vi "Main.vi"(11 "Module Admin":refnum<class "Delacor_lib_QMH_Module Admin.lvclass">) -> ()   [LabVIEW 2024, in "FunctionGenerator.lvlib"]
doc: "This template is based off of the Queued Message Handler design pattern and the Queued Message Handler project template that ships with LabVIEW.\n\nThe main difference is that the queue is private to this module and communication between modules is performed via Broadcast and Request events.\n\nRequest events are wrapped in public API methods and are handled in the Event Handling Loop (EHL) of this VI. Any module can register for Broadcast events sent by this module. The EHL generates messages based on user interface actions.\n\nThe Message Handling Loop (MHL) processes messages generated by the EHL, or by other messages. The messages are string values, so new messages can be added easily to the Message Cases case structure in the MHL. Each message cluster can also provide an optional value for Message Data, which is a variant that can be converted to whatever message-specific data is required.\n_____\nBased on DQMH Dev Tools: Project Template 7.1.0.1503."
uses:
  FunctionGenerator.lvlib
  <vilib>/Delacor/Delacor QMH/Libraries/Module Admin_class/Delacor_lib_QMH_Module Admin.lvclass
  Module Data--cluster.ctl
  <vilib>/Delacor/Delacor QMH/Libraries/Message Queue_class/Delacor_lib_QMH_Message Queue.lvclass/Delacor_lib_QMH_Message Queue.ctl
  Stop Argument--cluster.ctl
  <vilib>/Delacor/Delacor QMH/Libraries/Module Admin_class/Delacor_lib_QMH_Module Admin.lvclass/Delacor_lib_QMH_Module Admin.ctl
  Set Signal Type Argument--cluster.ctl
  Set Amplitude Argument--cluster.ctl
  Set Frecuency Argument--cluster.ctl
  Set Offset Argument--cluster.ctl
  Get Waveform Argument--cluster.ctl
  Get Waveform (Reply Payload)--cluster.ctl
  <vilib>/Utility/miscctls.llb/LVPointTypeDef.ctl
  <vilib>/Delacor/Delacor QMH/Libraries/Message Queue_class/Delacor_lib_QMH_Enqueue Message (Single).vi
  <vilib>/Delacor/Delacor QMH/Libraries/Module Admin_class/Delacor_lib_QMH_Get External Launch.vi
  <vilib>/Delacor/Delacor QMH/Libraries/Message Queue_class/Delacor_lib_QMH_Message Queue.lvclass
  <vilib>/measure/NI_MABase.lvlib
panel:
  out "error out":errorcluster
  out "Status":string
  in  "Simulate MHL Error":bool
  in  "Simulate EHL Error":bool
  # "Other processes communicate with this Module via its Public API (wrappers for its Request Events).\n\nThis Module communicates with other processes via its Broadcast Events.\nAny process that wants to receive these messages can register for this module's Broadcast events."
  # "This template is for the DQMH framework. See the block diagram for more information on how to use this template."
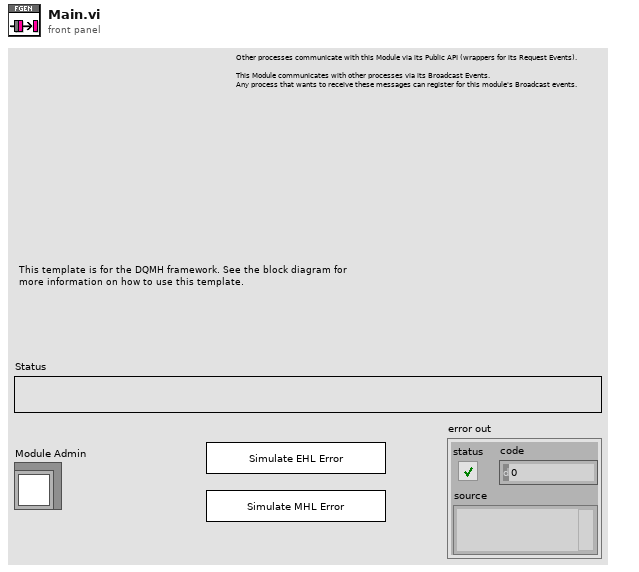
[diagram p1: front panel]
types:
  T1 = typedef "FunctionGenerator.lvlib/Request Events--cluster.ctl" = cluster{"Stop Module":refnum<user-event>, "Show Panel":refnum<user-event>, "Hide Panel":refnum<user-event>, "Get Module Execution Status":refnum<user-event>, "Show Diagram":refnum<user-event>, "Set Signal Type":refnum<user-event>, "Set Amplitude":refnum<user-event>, "Set Frecuency":refnum<user-event>, "Set Offset":refnum<user-event>, "Get Waveform":refnum<user-event>}
  T2 = typedef "FunctionGenerator.lvlib/Module Data--cluster.ctl" = cluster{"Status":string, "signal type":enum16{"Sine Wave", "Triangle Wave", "Square Wave", "Sawtooth Wave"}, "Amplitude":dbl, "Frecuency":dbl, "Offset":dbl}
  T3 = enum32{"invalid lock state", "Not Locked", "Locked (No Password)", "Password-protected"}
  T4 = typedef "FunctionGenerator.lvlib/Stop Argument--cluster.ctl" = cluster{"Origin":string, "Exit via Stop Module Req?":bool, "Wait for Module to stop?":bool}
  T5 = typedef "FunctionGenerator.lvlib/Set Signal Type Argument--cluster.ctl" = cluster{"signal type":enum16{"Sine Wave", "Triangle Wave", "Square Wave", "Sawtooth Wave"}}
  T6 = typedef "FunctionGenerator.lvlib/Set Amplitude Argument--cluster.ctl" = cluster{"Amplitude":dbl}
  T7 = typedef "FunctionGenerator.lvlib/Set Frecuency Argument--cluster.ctl" = cluster{"Frecuency":dbl}
  T8 = typedef "FunctionGenerator.lvlib/Set Offset Argument--cluster.ctl" = cluster{"Offset":dbl}
  T9 = typedef "FunctionGenerator.lvlib/Get Waveform Argument--cluster.ctl" = cluster{"Wait Notifier":refnum<notifier>, "wait for reply":bool}
  T10 = typedef "LVPointTypeDef.ctl" = cluster{"Horizontal":i16, "Vertical":i16}
  T11 = enum32{"Invalid", "Standard", "Closed", "Hidden", "Minimized", "Maximized"}
  T12 = typedef "FunctionGenerator.lvlib/Get Waveform (Reply Payload)--cluster.ctl" = cluster{"Waveform":waveform(dbl), "error":errorcluster}
  T13 = enum16{"Sine Wave", "Triangle Wave", "Square Wave", "Sawtooth Wave"}
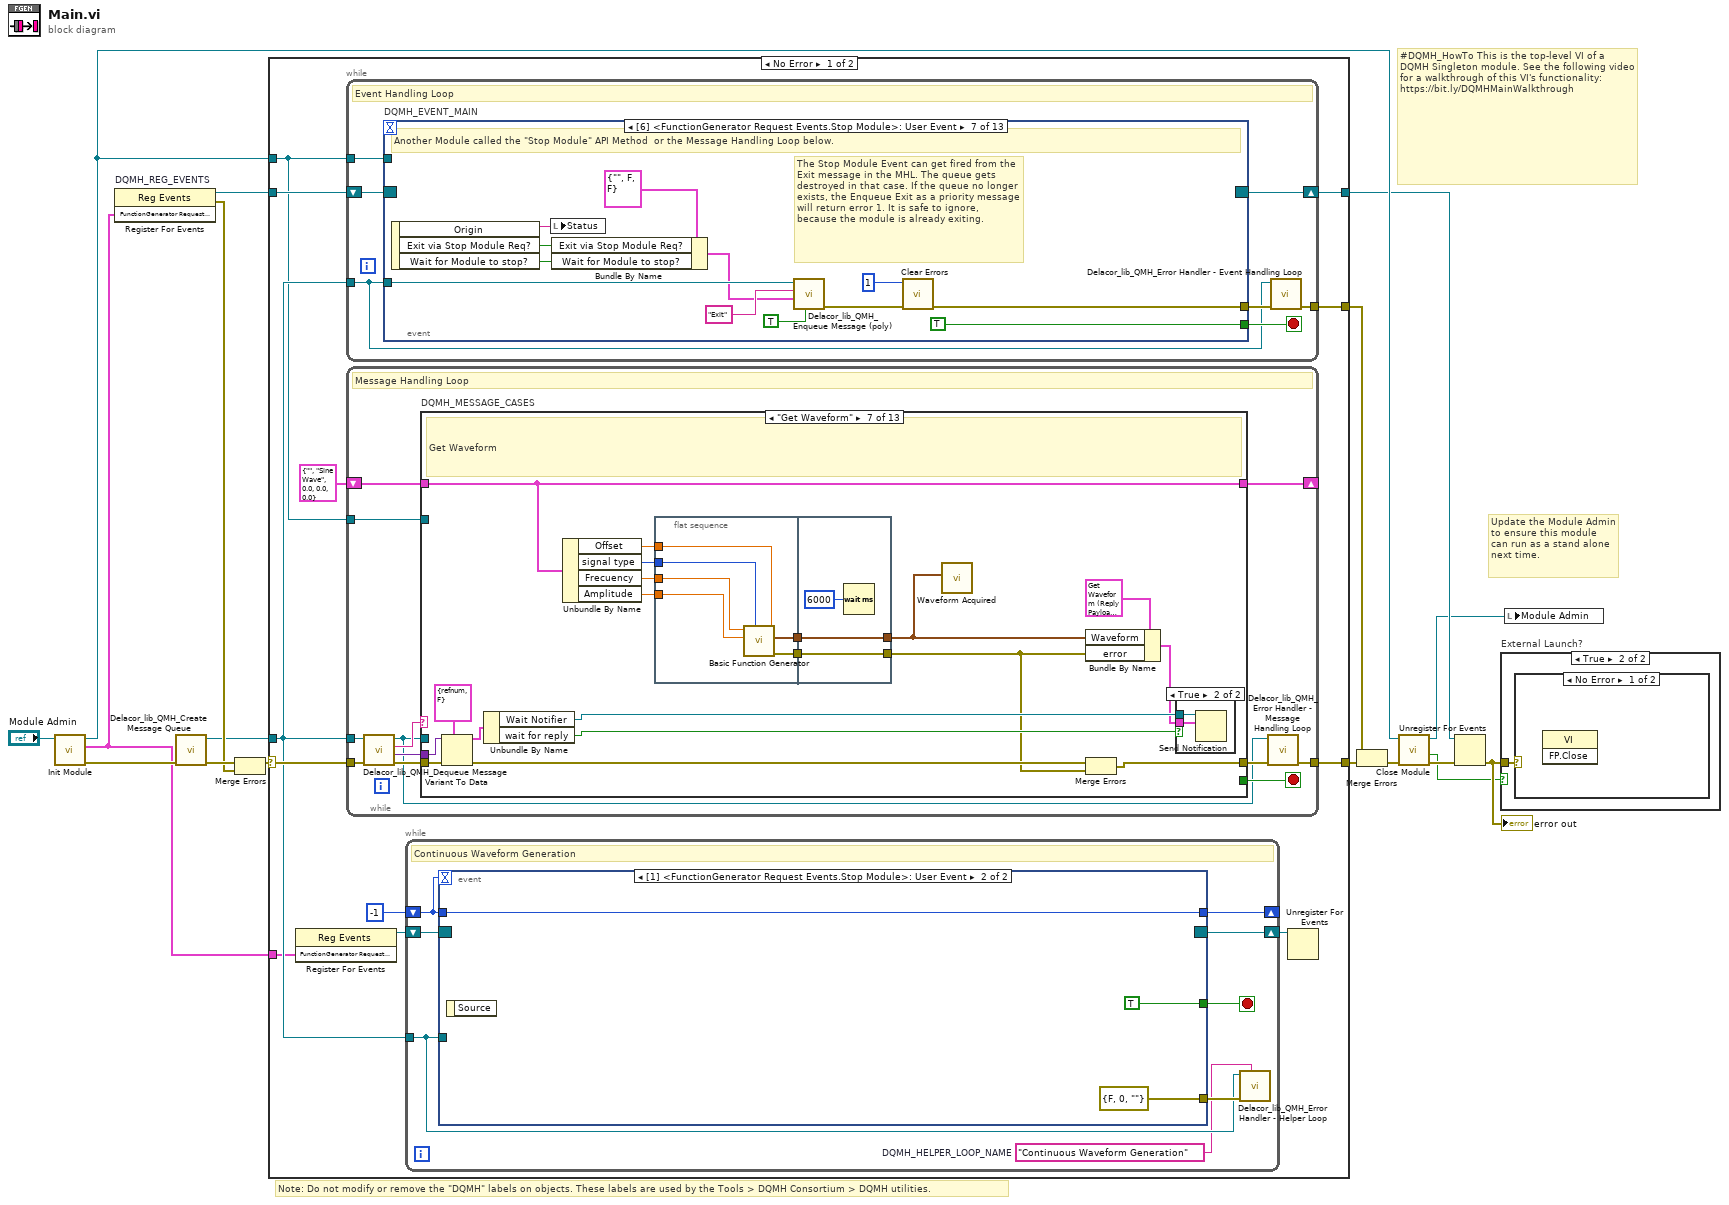
[diagram p0: block diagram]
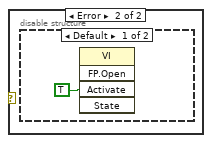
[diagram p3: hidden frame]
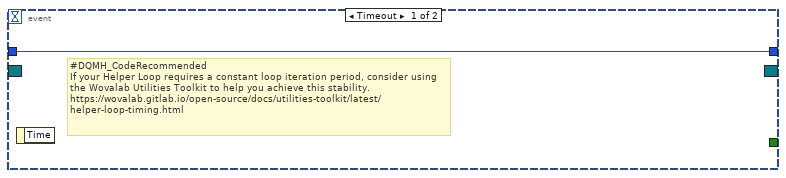
[diagram p5: hidden frame]
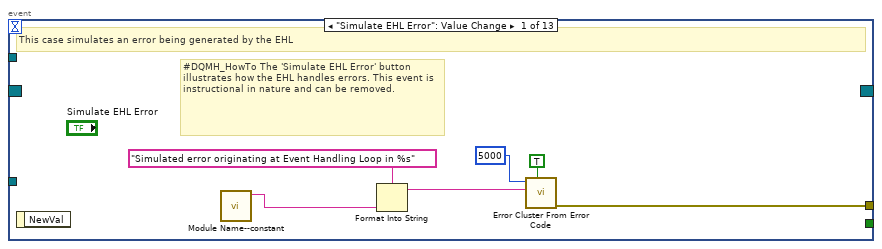
[diagram p6: hidden frame]
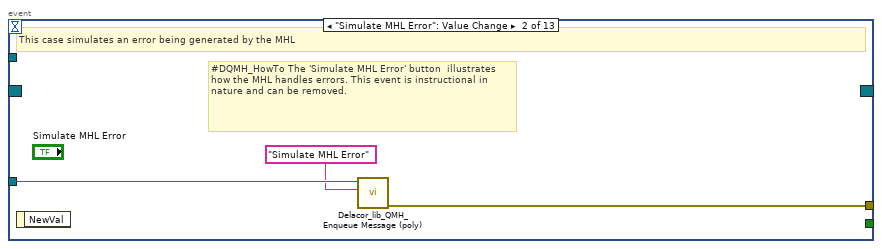
[diagram p7: hidden frame]
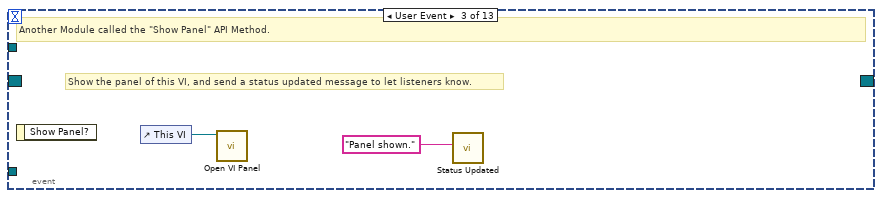
[diagram p8: hidden frame]
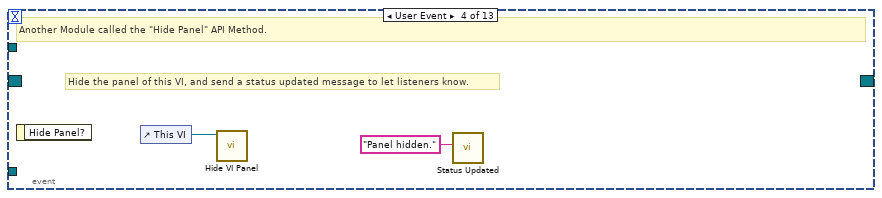
[diagram p9: hidden frame]
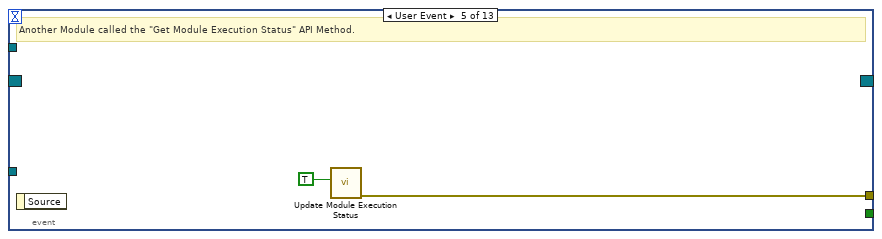
[diagram p10: hidden frame]
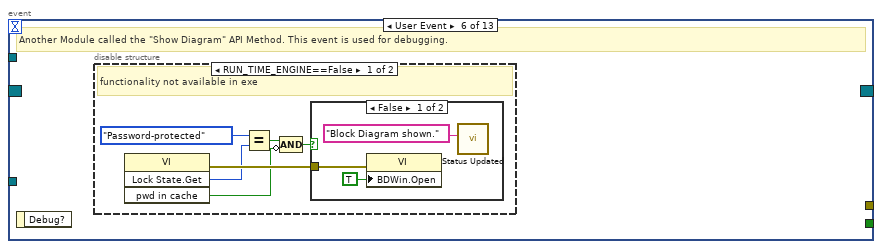
[diagram p11: hidden frame]
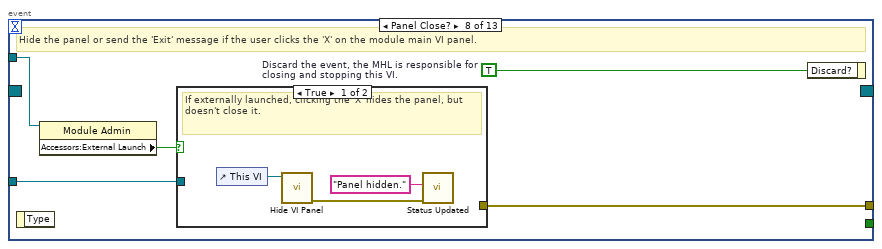
[diagram p14: hidden frame]
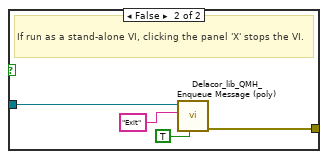
[diagram p15: hidden frame]
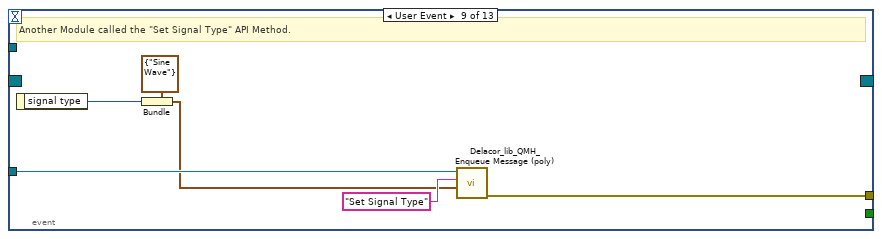
[diagram p16: hidden frame]
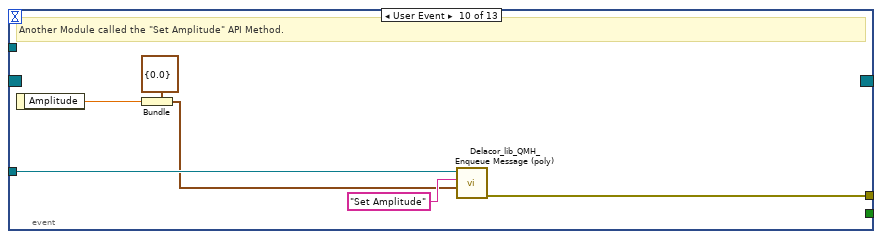
[diagram p17: hidden frame]
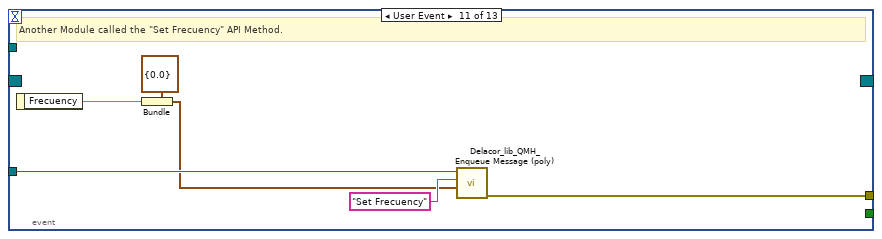
[diagram p18: hidden frame]
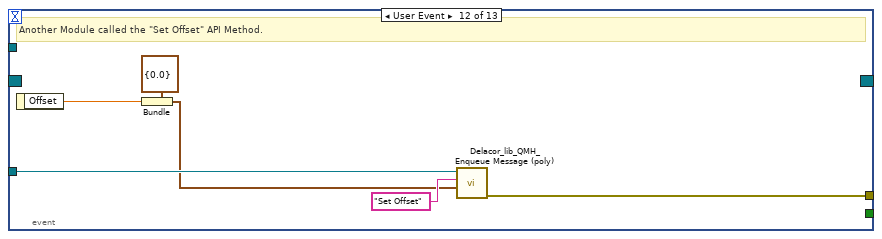
[diagram p19: hidden frame]
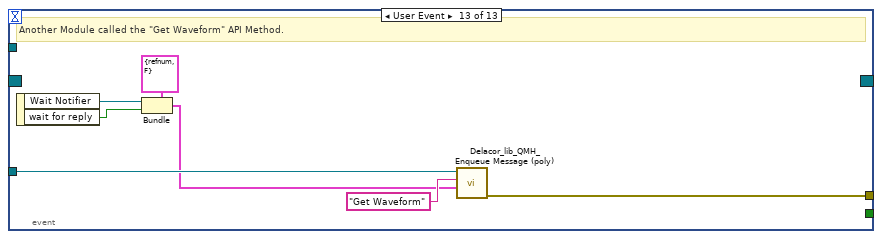
[diagram p20: hidden frame]
diagram:
  # "#DQMH_HowTo This is the top-level VI of a DQMH Singleton module. See the following video for a walkthrough of this VI's functionality: https://bit.ly/DQMHMainWalkthrough"
  # "Note: Do not modify or remove the \"DQMH\" labels on objects. These labels are used by the Tools > DQMH Consortium > DQMH utilities."
  # "Update the Module Admin to ensure this module can run as a stand alone next time."
  n1 = call "Init Module.vi"("Singleton Module Admin in"="Module Admin") -> ("error out"=w16:errorcluster, "FunctionGenerator Request Events"=w1:T1, "Singleton Module Admin out"=w8:refnum<class "Delacor_lib_QMH_Module Admin.lvclass">)  [unwired: 8 in]
  n2 = register-events "DQMH_REG_EVENTS"(w1) -> (reference out=w6:refnum<event-registration>, error out=w9:errorcluster)  [unwired: 2 in]
  n3 = call <vilib>:"Delacor_lib_QMH_Create Message Queue.vi"("error in"=w16) -> ("error out"=w11:errorcluster, "Message Queue"=w5:refnum<class "Delacor_lib_QMH_Message Queue.lvclass">)  [unwired: 9 in]
  n4 = Merge Errors(w11, w9) -> (w10:errorcluster)
  n5 = case shown="No Error" w10 {
    selector: w10 -> [w27 w295]
    tunnel: [w29 w294] -> w17
    tunnel: [w26 w293] -> w7
    tunnel: w6 -> [w24 w293]
    tunnel: w5 -> [w23 w288]
    tunnel: [w28 _] -> w14
    tunnel: w8 -> [w22 w289]
    tunnel: w1 -> [w21 _]
    frame No Error {
      n6 = register-events ("DQMH_HELPER_REGFOREVENTS")(w21) -> (reference out=w19:refnum<event-registration>)  [unwired: 2 in, 1 out]
      n7 = while {
        tunnel: w23 -> [w42]
        shift-right: [w45] -> w26
        shift-left: w24 -> [w46]
        tunnel: [w47] -> w28
        tunnel: w22 -> [w43]
        stop <- w44 stop-if-true
        # "Event Handling Loop"
        n8 = event "DQMH_EVENT_MAIN" shown="[6] <FunctionGenerator Request Events.Stop Module>: User Event" {
          selector: w46 -> [_ _ _ _ _ _ _ _ _ _ _ _ _]
          dyn-events: [_ _ _ _ _ _ _ _ _ _ _ _ _] -> w45
          timeout: _ -> [_ _ _ _ _ _ _ _ _ _ _ _ _]
          tunnel: [_ _ _ _ _ _ TRUE ("Discard?") _ _ _ _ _ _] -> w44
          tunnel: w42 -> [_ w56 _ _ _ _ w80 w87 w102 w108 w114 w120 w127]
          tunnel: [w54 w57 _ _ w63 _ w83 w89 w97 w103 w109 w115 w121] -> w48
          tunnel: w43 -> [_ _ _ _ _ _ _ w86 _ _ _ _ _]
          event "Simulate EHL Error": Value Change {
            # "#DQMH_HowTo The 'Simulate EHL Error' button  illustrates how the EHL handles errors. This event is instructional in nature and can be removed."
            # "This case simulates an error being generated by the EHL"
            n9 = event-data() -> ()  [unwired: 1 in, 1 out]
            n10 = call "Module Name--constant.vi"() -> ("Module Name"=w51:string)  [unwired: 11 in]
            n11 = Format Into String(format string="Simulated error originating at Event Handling Loop in %s", w51) -> (resulting string=w52:string)  [unwired: 2 in, 1 out]
            n12 = call <vilib>:"Error Cluster From Error Code.vi"("show call chain? (False)"=TRUE, "error message (\"\")"=w52, "error code (0)"=5000) -> ("error out"=w54:errorcluster)  [unwired: 6 in]
          }
          event "Simulate MHL Error": Value Change {
            # "#DQMH_HowTo The 'Simulate MHL Error' button  illustrates how the MHL handles errors. This event is instructional in nature and can be removed."
            # "This case simulates an error being generated by the MHL"
            n13 = event-data() -> ()  [unwired: 1 in, 1 out]
            n14 = call-poly <vilib>:"Delacor_lib_QMH_Enqueue Message (poly).vi"("Message"="Simulate MHL Error", "Message Queue in"=w56) -> ("error out"=w57:errorcluster)  [unwired: 8 in, 1 out]
          }
          event User Event {
            # "Show the panel of this VI, and send a status updated message to let listeners know."
            # "Another Module called the \"Show Panel\" API Method."
            n15 = event-data() -> ()  [unwired: 1 in, 1 out]
            n16 = control-ref of="This VI"() -> (w59:refnum<vi>)
            n17 = call "Open VI Panel.vi"("VI"=w59) -> ()  [unwired: 10 in, 1 out]
            n18 = call "Status Updated.vi"("Status"="Panel shown." ("format string")) -> ()  [unwired: 10 in, 1 out]
          }
          event User Event {
            # "Hide the panel of this VI, and send a status updated message to let listeners know."
            # "Another Module called the \"Hide Panel\" API Method."
            n19 = event-data() -> ()  [unwired: 1 in, 1 out]
            n20 = control-ref of="This VI"() -> (w61:refnum<vi>)
            n21 = call "Hide VI Panel.vi"("VI"=w61) -> ()  [unwired: 10 in, 1 out]
            n22 = call "Status Updated.vi"("Status"="Panel hidden." ("format string")) -> ()  [unwired: 10 in, 1 out]
          }
          event User Event {
            # "Another Module called the \"Get Module Execution Status\" API Method."
            n23 = event-data() -> ()  [unwired: 1 in, 1 out]
            n24 = call "Update Module Execution Status.vi"("Running?"=TRUE) -> ("error out"=w63:errorcluster)  [unwired: 10 in]
          }
          event User Event {
            # "Another Module called the \"Show Diagram\" API Method. This event is used for debugging."
            n25 = event-data() -> ()  [unwired: 1 in, 1 out]
            n26 = disable-structure shown="RUN_TIME_ENGINE==False" {
              frame condition #0 (active) {
                # "functionality not available in exe"
                n27 = invoke on="Invoke Node" class="VI" method="Lock State.Get"() -> (error out=w69:errorcluster, "Get Lock State"=w68:T3, "pwd in cache"=w65:bool)  [unwired: 4 in, 1 out]
                n28 = Equal?(x=T3."Password-protected", y=w68) -> (x = y?=w66:bool)
                n29 = Compound Arithmetic op=AND(w66, invert w65) -> (w64:bool)
                n30 = case shown="False" w64 {
                  tunnel: w69 -> [w72 _]
                  frame False {
                    n31 = property on="Property Node" class="VI"(error in=w72, "BDWin.Open"=TRUE ("Block Diagram Window:Open")) -> ()  [unwired: 1 in, 2 out]
                    n32 = call "Status Updated.vi"("Status"="Block Diagram shown." ("format string")) -> ()  [unwired: 10 in, 1 out]
                  }
                  frame True {
                    # "Password-protected VI, and the password is not in the cache. Do not show the diagram."
                  }
                }
              }
              frame condition #1 {
              }
            }
          }
          event User Event {
            # "The Stop Module Event can get fired from the Exit message in the MHL. The queue gets destroyed in that case. If the queue no longer exists, the Enqueue Exit as a priority message will return error 1. It is safe to ignore, because the module is already exiting."
            # "Another Module called the \"Stop Module\" API Method  or the Message Handling Loop below."
            n33 = event-data() -> ("Origin"=w79:string, "Exit via Stop Module Req?"=w75:bool, "Wait for Module to stop?"=w74:bool)  [unwired: 1 in]
            n34 = local write "Status"(w79) -> ()
            n35 = Bundle By Name(cluster=T4 {"Origin"="", "Exit via Stop Module Req?"=FALSE, "Wait for Module to stop?"=FALSE} ("Stop Argument"), "Exit via Stop Module Req?"=w75, "Wait for Module to stop?"=w74) -> (w73:T4)
            n36 = call-poly <vilib>:"Delacor_lib_QMH_Enqueue Message (poly).vi"("Priority Message? (F)"=TRUE, "Message Data"=w73, "Message"="Exit", "Message Queue in"=w80) -> ("error out"=w84:errorcluster)  [unwired: 6 in, 1 out]
            n37 = call <vilib>:"Clear Errors.vi"("error in (no error)"=w84, "specific error code to clear (0: all)"=1) -> ("error out"=w83:errorcluster)  [unwired: 4 in, 1 out]
          }
          event Panel Close? {
            w88 = TRUE  # Discard the event, the MHL is responsible for closing and stopping this VI.
            # "Hide the panel or send the 'Exit' message if the user clicks the 'X' on the module main VI panel."
            n38 = event-data() -> ()  [unwired: 1 in, 1 out]
            n39 = property on="Property Node" class="Module Admin"(reference=w86) -> ("Accessors:External Launch"=w85:bool)  [unwired: 1 in, 2 out]
            n40 = case shown="True" w85 {
              tunnel: w87 -> [_ w95]
              tunnel: [_ w96] -> w89
              frame True {
                # "If externally launched, clicking the 'X' hides the panel, but doesn't close it."
                n41 = control-ref of="This VI"() -> (w92:refnum<vi>)
                n42 = call "Hide VI Panel.vi"("VI"=w92) -> ("error out"=w90:errorcluster)  [unwired: 10 in]
                n43 = call "Status Updated.vi"("error in"=w90, "Status"="Panel hidden." ("format string")) -> ()  [unwired: 9 in, 1 out]
              }
              frame False {
                # "If run as a stand-alone VI, clicking the panel 'X' stops the VI."
                n44 = call-poly <vilib>:"Delacor_lib_QMH_Enqueue Message (poly).vi"("Priority Message? (F)"=TRUE, "Message"="Exit", "Message Queue in"=w95) -> ("error out"=w96:errorcluster)  [unwired: 7 in, 1 out]
              }
            }
            n45 = event-data ("Event Filter Node")("Discard?"=w88) -> ()  [unwired: 1 in, 1 out]
          }
          event User Event {
            # "Another Module called the \"Set Signal Type\" API Method."
            n46 = event-data() -> ("signal type"=w98:T13)  [unwired: 1 in]
            n47 = Bundle(cluster=T5 {"signal type"=enum."Sine Wave"} ("Set Signal Type Argument"), "signal type"=w98) -> (w99:T5)
            n48 = call-poly <vilib>:"Delacor_lib_QMH_Enqueue Message (poly).vi"("Message Data"=w99, "Message"="Set Signal Type", "Message Queue in"=w102) -> ("error out"=w97:errorcluster)  [unwired: 7 in, 1 out]
          }
          event User Event {
            # "Another Module called the \"Set Amplitude\" API Method."
            n49 = event-data() -> ("Amplitude"=w104:dbl)  [unwired: 1 in]
            n50 = Bundle(cluster=T6 {"Amplitude"=0.0} ("Set Amplitude Argument"), "Amplitude"=w104) -> (w105:T6)
            n51 = call-poly <vilib>:"Delacor_lib_QMH_Enqueue Message (poly).vi"("Message Data"=w105, "Message"="Set Amplitude", "Message Queue in"=w108) -> ("error out"=w103:errorcluster)  [unwired: 7 in, 1 out]
          }
          event User Event {
            # "Another Module called the \"Set Frecuency\" API Method."
            n52 = event-data() -> ("Frecuency"=w110:dbl)  [unwired: 1 in]
            n53 = Bundle(cluster=T7 {"Frecuency"=0.0} ("Set Frecuency Argument"), "Frecuency"=w110) -> (w111:T7)
            n54 = call-poly <vilib>:"Delacor_lib_QMH_Enqueue Message (poly).vi"("Message Data"=w111, "Message"="Set Frecuency", "Message Queue in"=w114) -> ("error out"=w109:errorcluster)  [unwired: 7 in, 1 out]
          }
          event User Event {
            # "Another Module called the \"Set Offset\" API Method."
            n55 = event-data() -> ("Offset"=w116:dbl)  [unwired: 1 in]
            n56 = Bundle(cluster=T8 {"Offset"=0.0} ("Set Offset Argument"), "Offset"=w116) -> (w117:T8)
            n57 = call-poly <vilib>:"Delacor_lib_QMH_Enqueue Message (poly).vi"("Message Data"=w117, "Message"="Set Offset", "Message Queue in"=w120) -> ("error out"=w115:errorcluster)  [unwired: 7 in, 1 out]
          }
          event User Event {
            # "Another Module called the \"Get Waveform\" API Method."
            n58 = event-data() -> ("Wait Notifier"=w123:refnum<notifier>, "wait for reply"=w122:bool)  [unwired: 1 in]
            n59 = Bundle(cluster=T9 {"Wait Notifier"=refnum, "wait for reply"=FALSE} ("Get Waveform Argument"), "Wait Notifier"=w123, "wait for reply"=w122) -> (w124:T9)
            n60 = call-poly <vilib>:"Delacor_lib_QMH_Enqueue Message (poly).vi"("Message Data"=w124, "Message"="Get Waveform", "Message Queue in"=w127) -> ("error out"=w121:errorcluster)  [unwired: 7 in, 1 out]
          }
        }
        n61 = call-dynamic "Delacor_lib_QMH_Error Handler - Event Handling Loop.vi"("error in"=w48, "Message Queue in"=w42) -> ("dup error in"=w47:errorcluster)  [unwired: 8 in, 1 out]
      }
      n62 = while {
        tunnel: w23 -> [w128]
        shift-right: [w136] -> _
        shift-left: T2 {"Status"="", "signal type"=enum."Sine Wave", "Amplitude"=0.0, "Frecuency"=0.0, "Offset"=0.0} ("Data Cluster") -> [w137]
        tunnel: w27 -> [w139]
        tunnel: [w131] -> w29
        tunnel: w22 -> [w132]
        stop <- w135 stop-if-true
        # "Message Handling Loop"
        n63 = call-dynamic "Delacor_lib_QMH_Dequeue Message.vi"("error in"=w139, "Message Queue in"=w128) -> ("error out"=w138:errorcluster, "Message Data"=w133:variant, "Message"=w134:string, "Message Queue out"=w129:refnum<class "Delacor_lib_QMH_Message Queue.lvclass">)  [unwired: 6 in]
        n64 = case "DQMH_MESSAGE_CASES" shown="\"Get Waveform\"" w134 {
          selector: w134 -> [_ _ _ _ _ _ _ _ _ _ _ _ w283]
          tunnel: w129 -> [_ _ _ _ _ _ _ _ _ _ w249 w271 _]
          tunnel: w138 -> [w157 w161 w171 w181 w191 w201 w220 w234 w236 w245 w256 w277 w286]
          tunnel: [w155 w161 w169 w179 w189 w199 w211 w233 w236 w244 w252 w272 w287] -> w130
          tunnel: w137 -> [w146 w160 w170 w180 w190 w200 w209 w232 w235 w242 w251 w270 w284]
          tunnel: [w145 w160 w165 w175 w183 w195 w209 w232 w235 w242 w251 w270 w284] -> w136
          tunnel: [_ _ _ _ _ _ _ _ _ _ _ w269 _] -> w135
          tunnel: w133 -> [_ _ w168 w178 w188 w198 w218 _ _ _ w250 w268 _]
          tunnel: w132 -> [w147 _ _ _ _ _ _ _ _ _ w248 w263 _]
          frame "Initialize" {
            w141 = "Initial Message" ("Initial Message")
            # "#DQMH_CodeNeeded - Initialize the appearance of the front panel."
            # "#DQMH_CodeNeeded - Initialize your state data here."
            # "Initialize - Any operation that needs to be done before the module can receive messages. Synchronize Caller Events.vi will inform Start Module.vi that the module has launched and is ready to receive messages. Module Did Init.vi will broadcast that the module initialized."
            n65 = call "Synchronize Caller Events.vi"("error in"=w157, "Singleton Module Admin in"=w147) -> ("error out"=w156:errorcluster, "Singleton Module Admin out"=w142:refnum<class "Delacor_lib_QMH_Module Admin.lvclass">)  [unwired: 8 in]
            n66 = property on="Property Node" class="Module Admin"(reference=w142) -> ("Accessors:External Launch"=w151:bool)  [unwired: 1 in, 2 out]
            n67 = Select(t=T11."Hidden" ("State"), s=w151, f=T11."Standard" ("State")) -> (s? t:f=w148:T11)
            n68 = call "Module Name--constant.vi"() -> ("Module Name"=w154:string)  [unwired: 11 in]
            n69 = property on="Property Node" class="VI"("Front Panel.Title"=w154) -> (reference out=w153:refnum<vi>, error out=w159:errorcluster)  [unwired: 2 in]
            n70 = invoke on="Invoke Node" class="VI" method="FP.Open"(reference=w153, error in=w159, "State"=w148) -> (reference out=w152:refnum<vi>, error out=w158:errorcluster)  [unwired: 2 in, 3 out]
            n71 = Bundle By Name(cluster=w146, "Status"=w141) -> (w145:T2)
            n72 = invoke on="Invoke Node" class="VI" method="FP.Center"(reference=w152, error in=w158) -> ()  [unwired: 1 in, 3 out]
            n73 = property on="Pane" class="Pane"("Origin"=T10 {"Horizontal"=0, "Vertical"=0}) -> ()  [unwired: 2 in, 2 out]
            n74 = call "Module Name--constant.vi"() -> ("Module Name"=w143:string)  [unwired: 11 in]
            n75 = call "Module Did Init.vi"("error in"=w156, "Initialized?"=TRUE, "Origin"=w143) -> ("error out"=w155:errorcluster)  [unwired: 8 in]
            "Status" <- w141
          }
          frame "---Module Specific---" {
            # "Separator -- The following cases handle messages specific to this Module."
          }
          frame "Set Signal Type" {
            # "Set Signal Type"
            n76 = Variant To Data(error in=w171, type=T5 {"signal type"=enum."Sine Wave"} ("Set Signal Type Argument"), Variant=w168) -> (data=w166:T5, error out=w169:errorcluster)
            n77 = Unbundle By Name(w166) -> ("signal type"=w163:T13)
            n78 = Bundle By Name(cluster=w170, "signal type"=w163) -> (w165:T2)
            n79 = Format Into String(format string="Signal type set to: %s", w163) -> (resulting string=w164:string)  [unwired: 2 in, 1 out]
            n80 = call "Status Updated.vi"("Status"=w164) -> ()  [unwired: 10 in, 1 out]
          }
          frame "Set Amplitude" {
            # "Set Amplitude"
            n81 = Variant To Data(error in=w181, type=T6 {"Amplitude"=0.0} ("Set Amplitude Argument"), Variant=w178) -> (data=w176:T6, error out=w179:errorcluster)
            n82 = Unbundle By Name(w176) -> ("Amplitude"=w174:dbl)
            n83 = Bundle By Name(cluster=w180, "Amplitude"=w174) -> (w175:T2)
            n84 = Format Into String(format string="Set Amplitude: %.2f", w174) -> (resulting string=w173:string)  [unwired: 2 in, 1 out]
            n85 = call "Status Updated.vi"("Status"=w173) -> ()  [unwired: 10 in, 1 out]
          }
          frame "Set Frecuency" {
            # "Set Frecuency"
            n86 = Variant To Data(error in=w191, type=T7 {"Frecuency"=0.0} ("Set Frecuency Argument"), Variant=w188) -> (data=w186:T7, error out=w189:errorcluster)
            n87 = Unbundle By Name(w186) -> ("Frecuency"=w182:dbl)
            n88 = Bundle By Name(cluster=w190, "Frecuency"=w182) -> (w183:T2)
            n89 = Format Into String(format string="Set Frecuency: %.2f", w182) -> (resulting string=w185:string)  [unwired: 2 in, 1 out]
            n90 = call "Status Updated.vi"("Status"=w185) -> ()  [unwired: 10 in, 1 out]
          }
          frame "Set Offset" {
            # "Set Offset"
            n91 = Variant To Data(error in=w201, type=T8 {"Offset"=0.0} ("Set Offset Argument"), Variant=w198) -> (data=w196:T8, error out=w199:errorcluster)
            n92 = Unbundle By Name(w196) -> ("Offset"=w192:dbl)
            n93 = Bundle By Name(cluster=w200, "Offset"=w192) -> (w195:T2)
            n94 = Format Into String(format string="Set Offset: %.2f", w192) -> (resulting string=w194:string)  [unwired: 2 in, 1 out]
            n95 = call "Status Updated.vi"("Status"=w194) -> ()  [unwired: 10 in, 1 out]
          }
          frame "Get Waveform" {
            # "Get Waveform"
            n96 = Variant To Data(error in=w220, type=T9 {"Wait Notifier"=refnum, "wait for reply"=FALSE} ("Get Waveform Argument"), Variant=w218) -> (data=w216:T9, error out=w219:errorcluster)
            n97 = Unbundle By Name(w216) -> ("Wait Notifier"=w215:refnum<notifier>, "wait for reply"=w214:bool)
            n98 = Unbundle By Name(w209) -> ("Offset"=w207:dbl, "signal type"=w208:T13, "Frecuency"=w206:dbl, "Amplitude"=w205:dbl)
            n99 = flat-sequence {
              tunnel: w208 -> [w225]
              tunnel: w207 -> [w224]
              tunnel: w206 -> [w223]
              tunnel: w205 -> [w222]
              tunnel: [w226] -> w203
              tunnel: [w221] -> w202
              tunnel: [w228] -> w204
              tunnel: [w229] -> w210
              tunnel: w203 -> [w229]
              tunnel: w202 -> [w228]
              frame #0 {
                n100 = call <vilib>:"Basic Function Generator.vi"("offset"=w224, "signal type"=w225, "amplitude"=w222, "frequency"=w223) -> ("error out"=w226:errorcluster, "signal out"=w221:waveform(dbl))  [unwired: 5 in, 1 out]
              }
              frame #1 {
                n101 = Wait (ms)(milliseconds to wait=u32 6000) -> ()  [unwired: 1 out]
              }
            }
            n102 = call "Waveform Acquired.vi"("Waveform"=w204) -> ()  [unwired: 10 in, 1 out]
            n103 = Bundle By Name(cluster=T12 {"Waveform"={"t0"=timestamp(0 s since 1904-01-01), "dt"=1.0, "Y"=[]}, "error"={"status"=FALSE, "code"=0, "source"=""}} ("Get Waveform (Reply Payload)"), "Waveform"=w204, "error"=w210) -> (w213:T12)
            n104 = Merge Errors(w219, w210) -> (w211:errorcluster)
            n105 = case "DQMH_FIRE_NOTIFIER" shown="True" w214 {
              tunnel: w215 -> [_ w231]
              tunnel: w213 -> [_ w230]
              frame False {
              }
              frame True {
                n106 = Send Notification(notification=w230, notifier=w231) -> ()  [unwired: 1 in, 2 out]
              }
            }
          }
          frame "---Copy This Frame---" {
            # "Duplicate this frame when creating new messages.  Change this comment in the duplicated frame to describe this message."
            n107 = Merge Errors(w234) -> (w233:errorcluster)
          }
          frame "---Exit and Error Handling---" {
            # "Separator - The following cases handle errors and exit messages."
          }
          frame "Simulate MHL Error" {
            # "#DQMH_HowTo The 'Simulate MHL Error' button  illustrates how the MHL handles errors. This event is instructional in nature and can be removed."
            # "Simulate an error occurring at the MHL"
            n108 = call "Module Name--constant.vi"() -> ("Module Name"=w238:string)  [unwired: 11 in]
            n109 = Format Into String(format string="Simulated error originating at Message Handling Loop in %s", w238) -> (resulting string=w239:string)  [unwired: 2 in, 1 out]
            n110 = call <vilib>:"Error Cluster From Error Code.vi"("show call chain? (False)"=TRUE, "error message (\"\")"=w239, "error code (0)"=5001) -> ("error out"=w243:errorcluster)  [unwired: 6 in]
            n111 = Merge Errors(w245, w243) -> (w244:errorcluster)
          }
          frame "Error" {
            # "#DQMH_CodeRecommended - If the module is running in standalone mode (External Launch = FALSE), this code will pop up an error dialog and call the 'Exit' message if an error occurs. Add more fine-grained error management here."
            # "Error - Check the error message data and respond accordingly. This message is sent by the \"Error Handler\" VIs at the end of each loop in this application."
            n112 = property on="Property Node" class="Module Admin"(reference=w248) -> ("Accessors:External Launch"=w247:bool)  [unwired: 1 in, 2 out]
            n113 = Variant To Data(error in=w256, type=errorcluster {"status"=FALSE, "code"=0, "source"=""} ("error constant"), Variant=w250) -> (data=w246:errorcluster, error out=w254:errorcluster)
            n114 = local write "error out"(w246) -> ()
            n115 = call "Error Reported.vi"("Error"=w246) -> ()  [unwired: 10 in, 1 out]
            n116 = case shown="False" w247 {
              tunnel: [w261 _] -> w253
              tunnel: w249 -> [w259 _]
              tunnel: w246 -> [w260 _]
              frame False {
                n117 = disable-structure shown="Default" {
                  disable-tunnel: w260 -> [w262 _]
                  frame condition #0 (active) {
                    # "If the module is running standalone, then pop up an error dialog and call the \"Exit\" message."
                    n118 = call <vilib>:"Simple Error Handler.vi"("error in (no error)"=w262) -> ()  [unwired: 4 in, 5 out]
                  }
                  frame condition #1 {
                    # "To prevent the Simple Error Handler VI from being loaded (e.g. when deploying to a Real-Time target), add the Conditional Disable Symbol \"DQMH_Disable_SEH\" to your project and set it to TRUE."
                  }
                }
                n119 = call-poly <vilib>:"Delacor_lib_QMH_Enqueue Message (poly).vi"("Priority Message? (F)"=TRUE, "Message"="Exit", "Message Queue in"=w259) -> ("error out"=w261:errorcluster)  [unwired: 7 in, 1 out]
              }
              frame True {
                # "If the module was launched externally, calling the Error Reported broadcast VI is the only action performed by the \"Error\" message. The module's caller can then process the error appropriately."
              }
            }
            n120 = Merge Errors(w254, w253) -> (w252:errorcluster)
          }
          frame "Exit" {
            w267 = 91  # 91: not all Exit messages will have an argument
            w269 = TRUE  # Stop the VI
            # "Release the message queue reference"
            # "#DQMH_CodeNeeded - Add any required cleanup code here."
            # "Exit - Exit the application."
            n121 = Variant To Data(error in=w277, type=T4 {"Origin"="", "Exit via Stop Module Req?"=FALSE, "Wait for Module to stop?"=FALSE} ("Stop Argument"), Variant=w268) -> (data=w265:T4, error out=w274:errorcluster)
            n122 = call <vilib>:"Clear Errors.vi"("error in (no error)"=w274, "specific error code to clear (0: all)"=w267) -> ("error out"=w276:errorcluster)  [unwired: 4 in, 1 out]
            n123 = control-ref of="This VI"() -> (w264:refnum<vi>)
            n124 = call-dynamic "Delacor_lib_QMH_Release Message Queue.vi"("error in"=w276, "Message Queue"=w271) -> ("error out"=w275:errorcluster)  [unwired: 9 in]
            n125 = call "Handle Exit.vi"("Stop Argument"=w265, "Admin in"=w263, "VI reference"=w264) -> ("error out"=w273:errorcluster)  [unwired: 7 in, 1 out]
            n126 = Merge Errors(w275, w273) -> (w272:errorcluster)
            n127 = call "Error Reported.vi"("Error"=w272) -> ()  [unwired: 10 in, 1 out]
          }
          frame Default {
            # "'Default' case only runs if there is a message that isn't defined in any of the other cases.  Output a programming error."
            n128 = call "Module Name--constant.vi"() -> ("Module Name"=w282:string)  [unwired: 11 in]
            n129 = Format Into String(format string="The invalid message string \"%s\" was received in the Message Handling Loop for module \"%s\".", w283, w282) -> (resulting string=w278:string)  [unwired: 2 in, 1 out]
            n130 = call <vilib>:"Error Cluster From Error Code.vi"("show call chain? (False)"=TRUE, "error message (\"\")"=w278, "error code (0)"=1) -> ("error out"=w285:errorcluster)  [unwired: 6 in]
            n131 = Merge Errors(w286, w285) -> (w287:errorcluster)
          }
        }
        n132 = call-dynamic "Delacor_lib_QMH_Error Handler - Message Handling Loop.vi"("error in"=w130, "Message Queue in"=w129) -> ("dup error in"=w131:errorcluster)  [unwired: 8 in, 1 out]
      }
      n133 = while "DQMH_HELPER_LOOP" {
        shift-right: [w37] -> _
        shift-left: -1 -> [w36]
        shift-right: [w34] -> w20
        shift-left: w19 -> [w35]
        tunnel: w23 -> [w31]
        stop <- w33 stop-if-true
        w30 = "Continuous Waveform Generation"  # DQMH_HELPER_LOOP_NAME
        # "Continuous Waveform Generation"
        n134 = event "DQMH_HELPER_EVENT_STRUCTURE" shown="[1] <FunctionGenerator Request Events.Stop Module>: User Event" {
          selector: w35 -> [_ _]
          dyn-events: [_ _] -> w34
          timeout: w36 -> [_ _]
          tunnel: w36 -> [w38 w41]
          tunnel: [w38 w41] -> w37
          tunnel: [_ TRUE] -> w33
          tunnel: [_ errorcluster {"status"=FALSE, "code"=0, "source"=""} ("error constant")] -> w32
          tunnel: w31 -> [_ _]
          event Timeout {
            # "#DQMH_CodeRecommended\nIf your Helper Loop requires a constant loop iteration period, consider using the Wovalab Utilities Toolkit to help you achieve this stability.\nhttps://wovalab.gitlab.io/open-source/docs/utilities-toolkit/latest/helper-loop-timing.html"
            n135 = event-data() -> ()  [unwired: 1 in, 1 out]
          }
          event User Event {
            n136 = event-data() -> ()  [unwired: 1 in, 1 out]
          }
        }
        n137 = call-dynamic "Delacor_lib_QMH_Error Handler - Helper Loop.vi"("Error Debug"=w30, "error in"=w32, "Message Queue in"=w31) -> ()  [unwired: 7 in, 2 out]
      }
      n138 = Unregister For Events(event registration refnum=w20) -> ()  [unwired: 1 in, 1 out]
    }
    frame Error {
      # "Synchronize Caller Events.vi will inform Start Module.vi that the module has launched and will let the code calling Start Module.vi register for broadcasts and would permit the caller receive the broadcast that an error occurred at launch time."
      n139 = call-dynamic "Delacor_lib_QMH_Release Message Queue.vi"("error in"=w295, "Message Queue"=w288) -> ("error out"=w294:errorcluster)  [unwired: 9 in]
      n140 = call "Synchronize Caller Events.vi"("Singleton Module Admin in"=w289) -> ("error out"=w296:errorcluster)  [unwired: 9 in, 1 out]
      n141 = call "Module Name--constant.vi"() -> ("Module Name"=w292:string)  [unwired: 11 in]
      n142 = Format Into String(format string="An error occurred during initialization. %s is no longer running.", w292) -> (resulting string=w290:string)  [unwired: 2 in, 1 out]
      n143 = Merge Errors(w294, w296) -> (w297:errorcluster)
      n144 = call "Error Reported.vi"("Additional Information"=w290, "Error"=w297) -> ()  [unwired: 9 in, 1 out]
    }
  }
  n145 = Merge Errors(w14, w17) -> (w13:errorcluster)
  n146 = call "Close Module.vi"("error in"=w13, "Module Admin in"=w8) -> ("error out"=w15:errorcluster, "External Launch"=w2:bool, "Module Admin out"=w3:refnum<class "Delacor_lib_QMH_Module Admin.lvclass">)  [unwired: 7 in]
  n147 = Unregister For Events(event registration refnum=w7, error in=w15) -> (error out=w12:errorcluster)
  "error out" <- w12
  n148 = case "External Launch?" shown="True" w2 {
    tunnel: w12 -> [_ w298]
    frame False {
    }
    frame True {
      n149 = case shown="No Error" w298 {
        frame No Error {
          n150 = invoke on="Invoke Node" class="VI" method="FP.Close"() -> ()  [unwired: 3 in, 3 out]
        }
        frame Error {
          n151 = disable-structure shown="Default" {
            frame condition #0 (active) {
              n152 = invoke class="VI" method="FP.Open"("Activate"=TRUE ("Activate?")) -> ()  [unwired: 4 in, 5 out]
            }
            frame condition #1 {
              # "Don't show panel on error if running inside a built EXE."
            }
          }
        }
      }
    }
  }
  n153 = local write "Module Admin"(w3) -> ()
